vi "Console_Queue.vi"(11 "Serial_Port":T3(xcontrol)) -> (1 "Queue out":refnum<queue>, 3 "Python":T1)   [LabVIEW 2022 SP3]
uses:
  Serial_Port.xctl
  PythonCtrl.ctl
  Processors.ctl
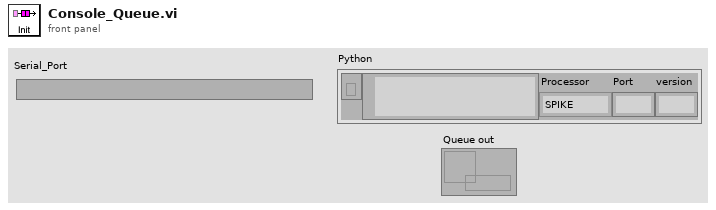
[diagram p1: front panel]
types:
  T1 = typedef "PythonCtrl.ctl" = cluster{"session":refnum<k35>, "PyPath":path, "Processor":T2, "Port":string, "version":string}
  T2 = typedef "Processors.ctl" = enum16{"SPIKE", "Pi", "Pi_ssh", "OpenMV", "Dunio"}
  T3 = cluster{"session":refnum<k35>, "PyPath":path, "Processor":T2, "Port":string, "version":string}
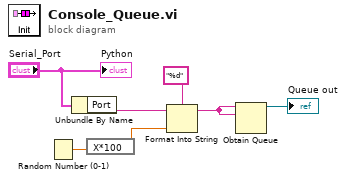
[diagram p0: block diagram]
diagram:
  n1 = Random Number (0-1)() -> (number: 0 to 1=w5:dbl)
  n2 = Unbundle By Name("Serial_Port") -> ("Port"=w3:string)
  n3 = expression code="X*100"(w5) -> (w4:dbl)
  n4 = Format Into String(format string="%d", initial string=w3, w4) -> (resulting string=w1:string)  [unwired: 1 in, 1 out]
  n5 = Obtain Queue(name (unnamed)=w1, element data type=w1) -> (queue out=→"Queue out":refnum<queue>)  [unwired: 3 in, 2 out]
  "Python" <- "Serial_Port"
